vi "T7_Write_UINT32_Register.vi"(8 "UINT32 to Write":u32, 9 "LabJack UINT32 Register":i32=55120, 10 "Remote Port":u16=502, 11 "Remote IP Address":string="192.168.1.15") -> ()   [LabVIEW 2017]
panel:
  # "MB Ethernet Example Master.vi\n\nInstructions\n1.Use Kipling to find your devices IP address & modify the\n\"Remote IP Addres\"\n2. Run this VI\n3. Change value of \"UINT32 to Write\" & press \"Write Data\""
  # "TCP Parameters"
  # "Test Write & Read of TEST_UINT32 Register"
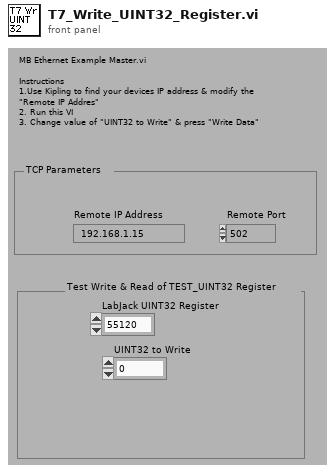
[diagram p1: front panel]
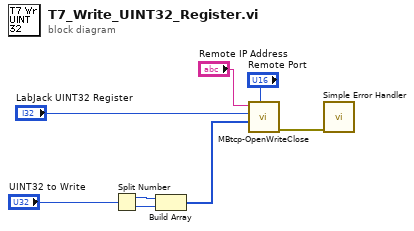
[diagram p0: block diagram]
diagram:
  n1 = Split Number(x="UINT32 to Write") -> (hi(x)=w7:u16, lo(x)=w6:u16)
  n2 = Build Array(w7, w6) -> (w2:u16[])
  n3 = call "MBtcp-OpenWriteClose.vi"("Port"="Remote Port", "Values"=w2, "RegisterAddr"="LabJack UINT32 Register", "IP Address"="Remote IP Address") -> ("error out"=w5:errorcluster)  [unwired: 7 in]
  n4 = call <vilib>:"Simple Error Handler.vi"("error in (no error)"=w5) -> ()  [unwired: 1 in, 8 out]
